vi "Begin.vi"(8 "error in":errorcluster) -> (0 "error out":errorcluster)   [LabVIEW 2018]
doc: "Called before other user functions, this VI is expected to open initial I/O refnums, load in file data, and do all program initialization. Notice that the <B>error out</B> terminal is simply used for data flow. Wiring it to other structures or subVIs ensures that this VI runs first."
uses:
  <vilib>/Rock Robotics/SystemInterfaces/DIO/FPGA_DIOPWMChannel.ctl
  <vilib>/Rock Robotics/WPI/DriverStation/WPI_DriverStationRobotMode2.ctl
  <vilib>/Rock Robotics/WPI/Joystick/WPI_JoystickDeviceEnum.ctl
  <vilib>/Rock Robotics/WPI/Solenoid/WPI_SolenoidChannel.ctl
  <vilib>/Rock Robotics/WPI/ThirdParty/REV Robotics/SPARK MAX/Typedef/Spark MAX Motor Type.ctl
  <vilib>/Rock Robotics/SystemInterfaces/DIO/FPGA_DIOChannel.ctl
  <vilib>/Rock Robotics/WPI/SafetyOutput/WPI_SafetyOutputConfigMenu.ctl
  <vilib>/Rock Robotics/WPI/ThirdParty/REV Robotics/SPARK MAX/Typedef/Spark MAX Idle Mode.ctl
  <vilib>/Rock Robotics/WPI/Solenoid/WPI_SolenoidValue.ctl
  Robot Global Data.vi
  <vilib>/Rock Robotics/Network Tables/NT Write String Array.vi
  <vilib>/Rock Robotics/WPI/Utilities/WPI_GetSetVariantRefNum.vi
  <vilib>/Rock Robotics/WPI/Counter/WPI_CounterDigitalInputToDigitalSource.vi
  <vilib>/Rock Robotics/WPI/MotorControl/WPI_MotorControlOpen SPARK.vi
  <vilib>/Rock Robotics/WPI/Solenoid/WPI_SolenoidOpenDouble.vi
  <vilib>/Rock Robotics/WPI/RobotDrive/WPI_RobotDriveOpen2MotorWithSPARK.vi
  <vilib>/Rock Robotics/WPI/RobotDrive/WPI_RobotDriveOpen4MotorWithSPARK.vi
  <vilib>/Rock Robotics/WPI/Switch/WPI_SwitchOpenLimit.vi
  <vilib>/Rock Robotics/WPI/Solenoid/WPI_SolenoidSetEnum.vi
  <vilib>/Rock Robotics/WPI/Ultrasonic/WPI_SonarSRF04DigitalOpen.vi
  <vilib>/Rock Robotics/WPI/Ultrasonic/WPI_SonarSRF04DigitalRefNum Registry Set.vi
  <vilib>/Rock Robotics/WPI/ThirdParty/REV Robotics/SPARK MAX/Typedef/Spark MAX Limit Switch Polarity.ctl
  <vilib>/Rock Robotics/WPI/ThirdParty/REV Robotics/SPARK MAX/Typedef/Spark MAX Limit Direction.ctl
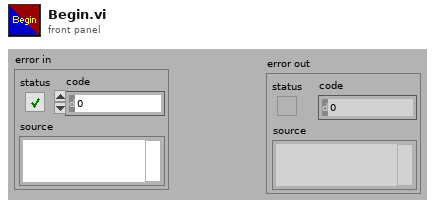
[diagram p1: front panel]
types:
  T1 = typedef "FPGA_DIOChannel.ctl" = enum8{"DIO 0", "DIO 1", "DIO 2", "DIO 3", "DIO 4", "DIO 5", "DIO 6", "DIO 7", "DIO 8", "DIO 9", "DIO MXP 0", "DIO MXP 1", "DIO MXP 2", "DIO MXP 3", "DIO MXP 4", "DIO MXP 5", "DIO MXP 6", "DIO MXP 7", "DIO MXP 8", "DIO MXP 9", "DIO MXP 10", "DIO MXP 11", "DIO MXP 12", "DIO MXP 13", "DIO MXP 14", "DIO MXP 15", "SPI Port CS1", "SPI Port CS2", "SPI Port CS3", "SPI Port MISO", "SPI Port MOSI", "Invalid"}
  T2 = typedef "WPI_SolenoidValue.ctl" = enum16{"Off", "On", "Forward", "Reverse"}
  T3 = typedef "WPI_SolenoidChannel.ctl" = enum8{"Solenoid 0", "Solenoid 1", "Solenoid 2", "Solenoid 3", "Solenoid 4", "Solenoid 5", "Solenoid 6", "Solenoid 7", "Invalid"}
  T4 = typedef "FPGA_DIOPWMChannel.ctl" = enum8{"PWM 0", "PWM 1", "PWM 2", "PWM 3", "PWM 4", "PWM 5", "PWM 6", "PWM 7", "PWM 8", "PWM 9", "PWM MXP 0", "PWM MXP 1", "PWM MXP 2", "PWM MXP 3", "PWM MXP 4", "PWM MXP 5", "PWM MXP 6", "PWM MXP 7", "PWM MXP 8", "PWM MXP 9", "Invalid"}
  T5 = typedef "Spark MAX Idle Mode.ctl" = enum16{"Coast", "Brake"}
  T6 = typedef "Spark MAX Motor Type.ctl" = enum16{"Brushed", "Brushless"}
  T7 = typedef "WPI_SafetyOutputConfigMenu.ctl" = enum16{"Enable", "Disable"}
  T8 = typedef "WPI_JoystickDeviceEnum.ctl" = enum16{"USB 0", "USB 1", "USB 2", "USB 3", "USB 4", "USB 5"}
  T9 = typedef "WPI_DriverStationRobotMode2.ctl" = enum16{"Autonomous Disabled", "Autonomous Enabled", "Teleop Disabled", "Teleop Enabled", "Disconnected", "Finish", "Test Disabled", "Test Enabled", "Emergency Stopped"}
  T10 = typedef "WPI_JoystickDevRef.ctl" = cluster{"Device":T8}
  T11 = typedef "WPI_SolenoidDevRef.ctl" = cluster{"DevStatus":errorcluster, "Pneumatics Control Module":u8, "Forward Solenoid Channel":T3, "Reverse Solenoid Channel":T3}
  T12 = typedef "WPI_CompressorDevRef.ctl" = cluster{"DevStatus":errorcluster, "Pneumatics Control Module":u8}
  T13 = typedef "WPI_RobotDriveDevRef.ctl" = cluster{"DevStatus":errorcluster, "Motors[]":T14[], "Square Inputs":bool, "Max Output":dbl}
  T14 = typedef "WPI_MotorControlDeviceRef.ctl" = cluster{"DeviceStatus":errorcluster, "Type":T15, "PWM":cluster{"PWM Channel":T4, "DeadBand":T16}, "CAN":cluster{"Device Number":u8, "SetOutput VI Ref":variant, "GetOutput VI Ref":variant, "Enable VI Ref":variant, "Disable VI Ref":variant, "Data":variant}, "Invert":bool, "DIO PWM":cluster{"PWM \"Enable\" Channel":T4, "DIOChannel":T1, "PWM Rate":dbl}}
  T15 = typedef "WPI_MotorControlType.ctl" = enum16{"PWM", "CAN", "DIO PWM"}
  T16 = typedef "WPI_PWMDeadband.ctl" = cluster{"Name":string, "maxPositivePwm":i32, "minPositivePwm":i32, "centerPwm":i32, "maxNegativePwm":i32, "minNegativePwm":i32, "angularRange":u16}
  T17 = typedef "WPI_DigitalInputDevRef.ctl" = cluster{"DevStatus":errorcluster, "DIO Channel":T1}
  T18 = typedef "FPGA_CounterEncoderSourceConvertionLVSourceType.ctl" = cluster{"DevStatus":errorcluster, "AnalogTriggerMode?":bool, "DigitalMode":cluster{"DIO Channel":T19}, "AnalogTriggerMode":cluster{"AnalogTriggerIndex":T20, "OutputType":T21}}
  T19 = typedef "FPGA_DIODigitalSourceChannel.ctl" = enum8{"DIO 0", "DIO 1", "DIO 2", "DIO 3", "DIO 4", "DIO 5", "DIO 6", "DIO 7", "DIO 8", "DIO 9", "DIO MXP 0", "DIO MXP 1", "DIO MXP 2", "DIO MXP 3", "DIO MXP 4", "DIO MXP 5", "DIO MXP 6", "DIO MXP 7", "DIO MXP 8", "DIO MXP 9", "DIO MXP 10", "DIO MXP 11", "DIO MXP 12", "DIO MXP 13", "DIO MXP 14", "DIO MXP 15", "SPI Port CS1", "SPI Port CS2", "SPI Port CS3", "SPI Port MISO", "SPI Port MOSI", "Disabled"}
  T20 = typedef "FPGA_AnalogTriggerIndex.ctl" = enum8{"Trig 0", "Trig 1", "Trig 2", "Trig 3", "Trig 4", "Trig 5", "Trig 6", "Trig 7", "Invalid"}
  T21 = typedef "FPGA_AnalogTriggerOutType.ctl" = enum16{"InWindow", "TriggerState", "Rising", "Falling"}
  T22 = typedef "WPI_EncoderDevRef.ctl" = cluster{"DevStatus":errorcluster, "EncoderIndex":T23, "CounterIndex":T24, "DistancePerCount":dbl, "Decoding Type":T25}
  T23 = typedef "FPGA_EncoderIdx.ctl" = enum8{"Enc 0", "Enc 1", "Enc 2", "Enc 3", "Enc 4", "Enc 5", "Enc 6", "Enc 7", "Invalid"}
  T24 = typedef "FPGA_CounterCtrSystemIndex.ctl" = enum8{"Ctr 0", "Ctr 1", "Ctr 2", "Ctr 3", "Ctr 4", "Ctr 5", "Ctr 6", "Ctr 7", "Invalid"}
  T25 = typedef "WPI_EncoderType.ctl" = enum16{"1x", "2x", "4x"}
  T26 = typedef "WPI_UltrasonicDeviceRef.ctl" = cluster{"DevStatus":errorcluster, "Ping Channel":T1, "Echo Channel":T1, "CntIndex":T24}
  T27 = typedef "WPI_SwitchDevRef.ctl" = cluster{"DevStatus":errorcluster, "DIO Channel":T1, "CntIndex":T24, "Normally Closed":bool}
  T28 = typedef "Spark MAX Limit Direction.ctl" = enum16{"Forward Limit", "Reverse Limit"}
  T29 = typedef "Spark MAX Limit Switch Polarity.ctl" = enum16{"Normally Open", "Normally Closed"}
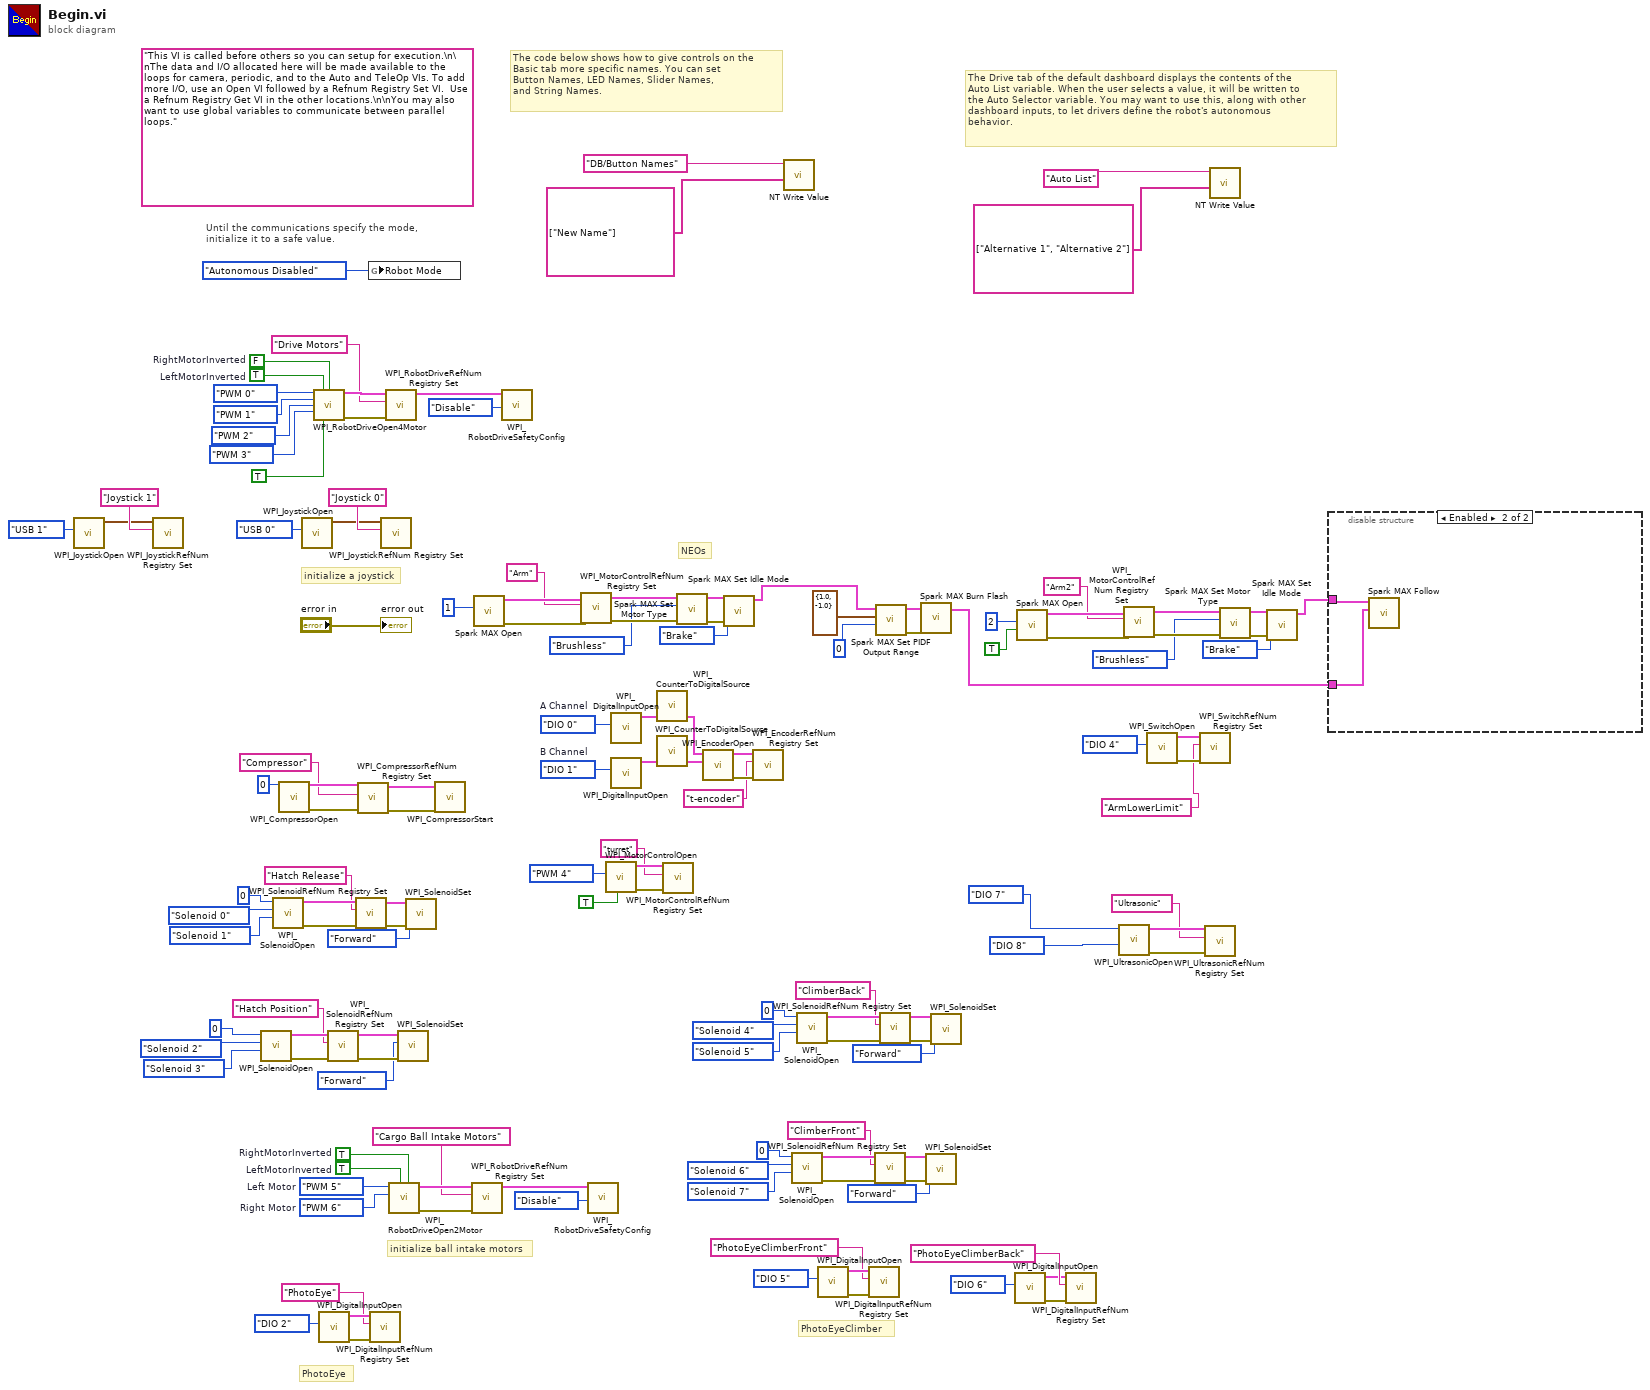
[diagram p0: block diagram]
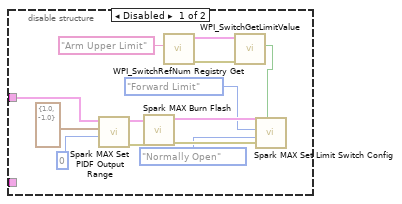
[diagram p2: hidden frame]
diagram:
  w64 = FPGA_DIOPWMChannel."PWM 6"  # Right Motor
  w65 = FPGA_DIOPWMChannel."PWM 5"  # Left Motor
  w69 = TRUE  # LeftMotorInverted
  w70 = TRUE  # RightMotorInverted
  w94 = FPGA_DIOChannel."DIO 1"  # B Channel
  w93 = FPGA_DIOChannel."DIO 0"  # A Channel
  (unwired) "This VI is called before others so you can setup for execution.\n\nThe data and I/O allocated here will be made available to the loops for camera, periodic, and to the Auto and TeleOp VIs. To add more I/O, use an Open VI followed by a Refnum Registry Set VI.  Use a Refnum Registry Get VI in the other locations.\n\nYou may also want to use global variables to communicate between parallel loops."
  w137 = TRUE  # LeftMotorInverted
  w138 = FALSE  # RightMotorInverted
  # "NEOs"
  # "PhotoEyeClimber"
  # "PhotoEye"
  # "initialize ball intake motors"
  # "The Drive tab of the default dashboard displays the contents of the\nAuto List variable. When the user selects a value, it will be written to\nthe Auto Selector variable. You may want to use this, along with other\ndashboard inputs, to let drivers define the robot's autonomous\nbehavior."
  # "The code below shows how to give controls on the\nBasic tab more specific names. You can set\nButton Names, LED Names, Slider Names,\nand String Names."
  # "initialize a joystick"
  # "Until the communications specify the mode,\ninitialize it to a safe value."
  n1 = call <vilib>:"WPI_JoystickOpen.vi"("JoystickDevice"=WPI_JoystickDeviceEnum."USB 1") -> ("JoystickDevRef"=w74:T10)  [unwired: 10 in]
  n2 = call <vilib>:"WPI_JoystickRefNum Registry Set.vi"("refnum name"="Joystick 1", "JoystickDevRef"=w74) -> ()  [unwired: 8 in, 2 out]
  n3 = call-poly <vilib>:"WPI_SolenoidOpen.vi"("Reverse Solenoid Channel"=WPI_SolenoidChannel."Solenoid 3", "Forward Solenoid Channel"=WPI_SolenoidChannel."Solenoid 2" ("Solenoid Channel"), "Pneumatics Control Module (0)"=u8 0) -> ("error out"=w79:errorcluster, "SolenoidDevRef"=w80:T11)  [unwired: 7 in]
  n4 = call-poly <vilib>:"WPI_SolenoidOpen.vi"("Reverse Solenoid Channel"=WPI_SolenoidChannel."Solenoid 1", "Forward Solenoid Channel"=WPI_SolenoidChannel."Solenoid 0" ("Solenoid Channel"), "Pneumatics Control Module (0)"=u8 0) -> ("error out"=w113:errorcluster, "SolenoidDevRef"=w114:T11)  [unwired: 7 in]
  n5 = call <vilib>:"WPI_CompressorOpen.vi"("Pneumatics Control Module (0)"=u8 0) -> ("CompressorDevRef"=w120:T12, "error out"=w119:errorcluster)  [unwired: 13 in]
  n6 = call <vilib>:"WPI_JoystickOpen.vi"("JoystickDevice"=WPI_JoystickDeviceEnum."USB 0") -> ("JoystickDevRef"=w127:T10)  [unwired: 10 in]
  n7 = call-poly <vilib>:"WPI_RobotDriveOpen4Motor.vi"("Rear Left Motor"=FPGA_DIOPWMChannel."PWM 0", "Rear Left Motor Inverted"=w137, "Rear Right Motor Inverted"=w138, "Rear Right Motor"=FPGA_DIOPWMChannel."PWM 1", "Front Left Motor"=FPGA_DIOPWMChannel."PWM 2", "Front Right Motor"=FPGA_DIOPWMChannel."PWM 3", "Front Left Motor Inverted"=TRUE) -> ("RobotDriveDevRef"=w136:T13, "error out"=w134:errorcluster)  [unwired: 7 in]
  n8 = call <vilib>:"WPI_DigitalInputOpen.vi"("DIO Channel"=FPGA_DIOChannel."DIO 2") -> ("error out"=w60:errorcluster, "DigitalInputDevRef"=w59:T17)  [unwired: 9 in]
  n9 = call <vilib>:"WPI_SolenoidRefNum Registry Set.vi"("error in (no error)"=w79, "refnum name"="Hatch Position", "SolenoidDevRef"=w80) -> ("error out"=w23:errorcluster, "SolenoidDevRef"=w24:T11)  [unwired: 7 in]
  n10 = call <vilib>:"WPI_SolenoidRefNum Registry Set.vi"("error in (no error)"=w113, "refnum name"="Hatch Release", "SolenoidDevRef"=w114) -> ("error out"=w26:errorcluster, "SolenoidDevRef"=w27:T11)  [unwired: 7 in]
  n11 = call <vilib>:"WPI_CompressorRefNum Registry Set.vi"("error in (no error)"=w119, "refnum name"="Compressor", "CompressorDevRef"=w120) -> ("error out"=w115:errorcluster, "CompressorDevRef"=w116:T12)  [unwired: 7 in]
  n12 = global write "Robot Global Data.vi" "Robot Mode"(WPI_DriverStationRobotMode2."Autonomous Disabled" ("Robot Mode")) -> ()
  n13 = call <vilib>:"WPI_DigitalInputRefNum Registry Set.vi"("error in (no error)"=w60, "refnum name"="PhotoEye", "DigitalInputDevRef"=w59) -> ()  [unwired: 7 in, 2 out]
  n14 = call <vilib>:"WPI_JoystickRefNum Registry Set.vi"("refnum name"="Joystick 0", "JoystickDevRef"=w127) -> ()  [unwired: 8 in, 2 out]
  n15 = call <vilib>:"WPI_RobotDriveRefNum Registry Set.vi"("error in (no error)"=w134, "refnum name"="Drive Motors", "RobotDriveDevRef"=w136) -> ("RobotDriveDevRef"=w131:T13)  [unwired: 1 in, 7 out]
  n16 = call-poly <vilib>:"WPI_RobotDriveOpen2Motor.vi"("Right Motor Inverted"=w70, "Left Motor Inverted"=w69, "Right Motor"=w64, "Left Motor"=w65) -> ("error out"=w66:errorcluster, "RobotDriveDevRef"=w68:T13)  [unwired: 1 in, 5 out]
  n17 = call-poly <vilib>:"WPI_SolenoidSet.vi"("error in (no error)"=w23, "Value"=WPI_SolenoidValue."Forward", "SolenoidDevRef"=w24) -> ()  [unwired: 7 in, 2 out]
  n18 = call-poly <vilib>:"WPI_SolenoidSet.vi"("error in (no error)"=w26, "Value"=WPI_SolenoidValue."Forward", "SolenoidDevRef"=w27) -> ()  [unwired: 7 in, 2 out]
  n19 = call <vilib>:"WPI_CompressorStart.vi"("error in (no error)"=w115, "CompressorDevRef"=w116) -> ()  [unwired: 8 in, 2 out]
  n20 = call <vilib>:"WPI_RobotDriveRefNum Registry Set.vi"("error in (no error)"=w66, "refnum name"="Cargo Ball Intake Motors", "RobotDriveDevRef"=w68) -> ("RobotDriveDevRef"=w63:T13)  [unwired: 1 in, 7 out]
  n21 = call <vilib>:"Spark MAX Open.vi"("Device Number"=u8 1) -> ("error out"=w107:errorcluster, "MotorControlDeviceRef"=w108:T14)  [unwired: 9 in]
  n22 = call <vilib>:"WPI_RobotDriveSafetyConfig.vi"("mode"=WPI_SafetyOutputConfigMenu."Disable", "RobotDriveDevRef"=w131) -> ()  [unwired: 8 in, 2 out]
  n23 = call <vilib>:"WPI_MotorControlRefNum Registry Set.vi"("error in (no error)"=w107, "refnum name"="Arm", "MotorControlDevRef"=w108) -> ("error out"=w104:errorcluster, "MotorControlDevRef"=w105:T14)  [unwired: 7 in]
  n24 = call <vilib>:"WPI_RobotDriveSafetyConfig.vi"("mode"=WPI_SafetyOutputConfigMenu."Disable", "RobotDriveDevRef"=w63) -> ()  [unwired: 8 in, 2 out]
  n25 = call-poly <vilib>:"WPI_MotorControlOpen.vi"("Invert"=TRUE, "PWM Channel"=FPGA_DIOPWMChannel."PWM 4") -> ("error out"=w84:errorcluster, "MotorControlDeviceRef"=w83:T14)  [unwired: 8 in]
  n26 = call <vilib>:"WPI_DigitalInputOpen.vi"("DIO Channel"=w93) -> ("DigitalInputDevRef"=w90:T17)  [unwired: 1 in, 9 out]
  n27 = call <vilib>:"WPI_DigitalInputOpen.vi"("DIO Channel"=w94) -> ("DigitalInputDevRef"=w91:T17)  [unwired: 1 in, 9 out]
  n28 = call-poly <vilib>:"WPI_CounterToDigitalSource.vi"("DigitalInputDevRef"=w90) -> ("Digital Source"=w89:T18)  [unwired: 6 out]
  n29 = call-poly <vilib>:"WPI_CounterToDigitalSource.vi"("DigitalInputDevRef"=w91) -> ("Digital Source"=w92:T18)  [unwired: 6 out]
  n30 = call <vilib>:"WPI_MotorControlRefNum Registry Set.vi"("error in (no error)"=w84, "refnum name"="turret", "MotorControlDevRef"=w83) -> ()  [unwired: 7 in, 2 out]
  n31 = call <vilib>:"Spark MAX Set Motor Type.vi"("error in (no error)"=w104, "Enum"=Spark_MAX_Motor_Type."Brushless", "MotorControlDevRef"=w105) -> ("error out"=w102:errorcluster, "MotorControlDeviceRef"=w101:T14)  [unwired: 7 in]
  n32 = call <vilib>:"WPI_EncoderOpen.vi"("BSource"=w92, "ASource"=w89) -> ("error out"=w88:errorcluster, "EncoderDevRef"=w87:T22)  [unwired: 6 in, 2 out]
  n33 = call <vilib>:"Spark MAX Set Idle Mode.vi"("error in (no error)"=w102, "Idle Mode"=Spark_MAX_Idle_Mode."Brake", "MotorControlDeviceRef in"=w101) -> ("MotorControlDeviceRef out"=w97:T14)  [unwired: 7 in, 1 out]
  n34 = call <vilib>:"WPI_EncoderRefNum Registry Set.vi"("error in (no error)"=w88, "refnum name"="t-encoder", "EncoderDevRef"=w87) -> ()  [unwired: 7 in, 2 out]
  n35 = call-poly <vilib>:"NT Write Value.vi"("String Array"=string[] ["New Name"], "Name"="DB/Button Names") -> ()  [unwired: 9 in, 1 out]
  n36 = call-poly <vilib>:"WPI_SolenoidOpen.vi"("Reverse Solenoid Channel"=WPI_SolenoidChannel."Solenoid 7", "Forward Solenoid Channel"=WPI_SolenoidChannel."Solenoid 6" ("Solenoid Channel"), "Pneumatics Control Module (0)"=u8 0) -> ("error out"=w17:errorcluster, "SolenoidDevRef"=w18:T11)  [unwired: 7 in]
  n37 = call-poly <vilib>:"WPI_SolenoidOpen.vi"("Reverse Solenoid Channel"=WPI_SolenoidChannel."Solenoid 5", "Forward Solenoid Channel"=WPI_SolenoidChannel."Solenoid 4" ("Solenoid Channel"), "Pneumatics Control Module (0)"=u8 0) -> ("error out"=w56:errorcluster, "SolenoidDevRef"=w57:T11)  [unwired: 7 in]
  n38 = call <vilib>:"WPI_DigitalInputOpen.vi"("DIO Channel"=FPGA_DIOChannel."DIO 5") -> ("error out"=w34:errorcluster, "DigitalInputDevRef"=w33:T17)  [unwired: 9 in]
  n39 = call <vilib>:"WPI_DigitalInputRefNum Registry Set.vi"("error in (no error)"=w34, "refnum name"="PhotoEyeClimberFront", "DigitalInputDevRef"=w33) -> ()  [unwired: 7 in, 2 out]
  n40 = call <vilib>:"WPI_SolenoidRefNum Registry Set.vi"("error in (no error)"=w17, "refnum name"="ClimberFront", "SolenoidDevRef"=w18) -> ("error out"=w11:errorcluster, "SolenoidDevRef"=w12:T11)  [unwired: 7 in]
  n41 = call <vilib>:"Spark MAX Set PIDF Output Range.vi"("PIDF Slot (0)"=0 ("PIDF Slot"), "output range"=cluster{"output max":dbl, "output min":dbl} {"output max"=1.0, "output min"=-1.0}, "MotorControlDeviceRef"=w97) -> ("error out"=w96:errorcluster, "MotorControlDeviceRef"=w95:T14)  [unwired: 7 in]
  n42 = call <vilib>:"WPI_SolenoidRefNum Registry Set.vi"("error in (no error)"=w56, "refnum name"="ClimberBack", "SolenoidDevRef"=w57) -> ("error out"=w20:errorcluster, "SolenoidDevRef"=w21:T11)  [unwired: 7 in]
  n43 = call <vilib>:"Spark MAX Burn Flash.vi"("error in"=w96, "MotorControlDeviceRef"=w95) -> ("MotorControlDeviceRef"=w38:T14)  [unwired: 8 in, 1 out]
  n44 = call-poly <vilib>:"WPI_SolenoidSet.vi"("error in (no error)"=w11, "Value"=WPI_SolenoidValue."Forward", "SolenoidDevRef"=w12) -> ()  [unwired: 7 in, 2 out]
  n45 = call-poly <vilib>:"WPI_SolenoidSet.vi"("error in (no error)"=w20, "Value"=WPI_SolenoidValue."Forward", "SolenoidDevRef"=w21) -> ()  [unwired: 7 in, 2 out]
  n46 = call <vilib>:"WPI_DigitalInputOpen.vi"("DIO Channel"=FPGA_DIOChannel."DIO 6") -> ("error out"=w7:errorcluster, "DigitalInputDevRef"=w8:T17)  [unwired: 9 in]
  n47 = call <vilib>:"Spark MAX Open.vi"("Invert"=TRUE, "Device Number"=u8 2) -> ("error out"=w51:errorcluster, "MotorControlDeviceRef"=w52:T14)  [unwired: 8 in]
  n48 = call <vilib>:"WPI_DigitalInputRefNum Registry Set.vi"("error in (no error)"=w7, "refnum name"="PhotoEyeClimberBack", "DigitalInputDevRef"=w8) -> ()  [unwired: 7 in, 2 out]
  n49 = call-poly <vilib>:"WPI_UltrasonicOpen.vi"("Echo DIO Channel"=FPGA_DIOChannel."DIO 8", "Ping DIO Channel"=FPGA_DIOChannel."DIO 7") -> ("error out"=w4:errorcluster, "SonarSRF04DevRef"=w5:T26)  [unwired: 8 in]
  n50 = call <vilib>:"WPI_MotorControlRefNum Registry Set.vi"("error in (no error)"=w51, "refnum name"="Arm2", "MotorControlDevRef"=w52) -> ("error out"=w48:errorcluster, "MotorControlDevRef"=w49:T14)  [unwired: 7 in]
  n51 = call-poly <vilib>:"WPI_SwitchOpen.vi"("DIO Channel"=FPGA_DIOChannel."DIO 4") -> ("error out"=w30:errorcluster, "SwitchDevRef"=w29:T27)  [unwired: 9 in]
  n52 = call <vilib>:"WPI_SwitchRefNum Registry Set.vi"("error in (no error)"=w30, "refnum name"="ArmLowerLimit", "SwitchDevRef"=w29) -> ()  [unwired: 7 in, 2 out]
  n53 = call-poly <vilib>:"WPI_UltrasonicRefNum Registry Set.vi"("error in (no error)"=w4, "refnum name"="Ultrasonic", "SonarSRF04DevRef"=w5) -> ()  [unwired: 7 in, 2 out]
  n54 = call-poly <vilib>:"NT Write Value.vi"("String Array"=string[] ["Alternative 1", "Alternative 2"], "Name"="Auto List") -> ()  [unwired: 9 in, 1 out]
  n55 = call <vilib>:"Spark MAX Set Motor Type.vi"("error in (no error)"=w48, "Enum"=Spark_MAX_Motor_Type."Brushless", "MotorControlDevRef"=w49) -> ("error out"=w46:errorcluster, "MotorControlDeviceRef"=w45:T14)  [unwired: 7 in]
  n56 = call <vilib>:"Spark MAX Set Idle Mode.vi"("error in (no error)"=w46, "Idle Mode"=Spark_MAX_Idle_Mode."Brake", "MotorControlDeviceRef in"=w45) -> ("MotorControlDeviceRef out"=w43:T14)  [unwired: 7 in, 1 out]
  n57 = disable-structure shown="Enabled" {
    disable-tunnel: w43 -> [w149 w152]
    disable-tunnel: w38 -> [_ w153]
    frame Disabled {
      n58 = call <vilib>:"Spark MAX Set PIDF Output Range.vi"("PIDF Slot (0)"=0 ("PIDF Slot"), "output range"=cluster{"output max":dbl, "output min":dbl} {"output max"=1.0, "output min"=-1.0}, "MotorControlDeviceRef"=w149) -> ("error out"=w148:errorcluster, "MotorControlDeviceRef"=w147:T14)  [unwired: 7 in]
      n59 = call <vilib>:"Spark MAX Burn Flash.vi"("error in"=w148, "MotorControlDeviceRef"=w147) -> ("error out"=w146:errorcluster, "MotorControlDeviceRef"=w145:T14)  [unwired: 8 in]
      n60 = call <vilib>:"WPI_SwitchRefNum Registry Get.vi"("refnum name"="Arm Upper Limit") -> ("error out"=w140:errorcluster, "SwitchDevRef"=w141:T27)  [unwired: 9 in]
      n61 = call <vilib>:"WPI_SwitchGetLimitValue.vi"("error in (no error)"=w140, "SwitchDevRef"=w141) -> ("Switch Pressed"=w142:bool)  [unwired: 7 in, 2 out]
      n62 = call <vilib>:"Spark MAX Set Limit Switch Config.vi"("Enabled? (T)"=w142, "error in (no error)"=w146, "Polarity (Normally Open)"=Spark_MAX_Limit_Switch_Polarity."Normally Open", "Limit Switch"=Spark_MAX_Limit_Direction."Forward Limit", "MotorControlDeviceRef in"=w145) -> ()  [unwired: 5 in, 2 out]
    }
    frame Enabled {
      n63 = call <vilib>:"Spark MAX Follow.vi"("Master Controller"=w153, "MotorControlDeviceRef"=w152) -> ()  [unwired: 8 in, 2 out]
    }
  }
  "error out" <- "error in"
